vi "test_advanced_Doppler_filtered.vi"() -> ()   [LabVIEW 2009]
doc: "Copyright (C) 2009, Stepan A. Baranov\nweb: http://www.OCTLab.org/\nemail: stepan@baranov.su"
uses:
  OCTLib.dll
panel:
  out "version":string
  out "name":string
  out "error out":errorcluster
  out "max":dbl
  out "min":dbl
  out "cell width":i32
  out "cell height":i32
  out "A-scan size":i32
  out "# of A-scans":i32
  in  "Small/Big":bool
  out "loop #":i32
  out "RSM_STAT time":u32
  out "LabView time":u32
  out "RSM_STAT Array":dbl[][](array[numeric])
  out "LabView Array":dbl[][](array[numeric])
  in  "stop":bool
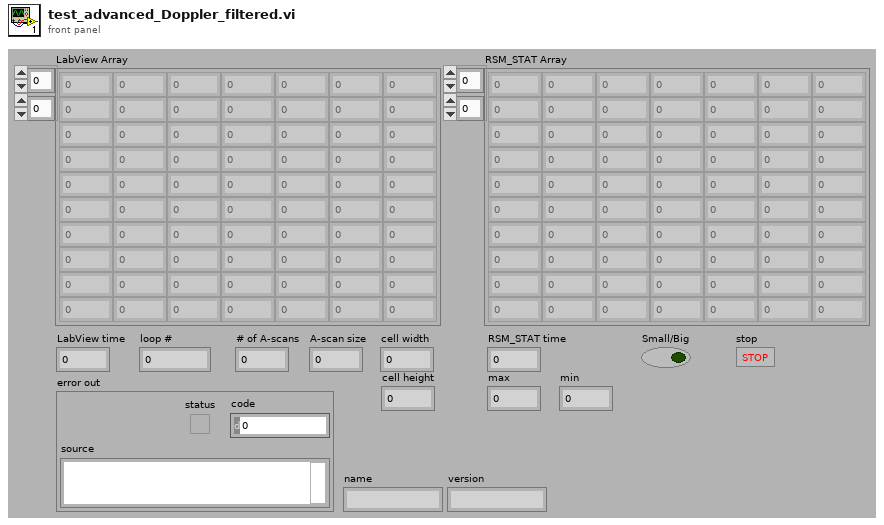
[diagram p1: front panel]
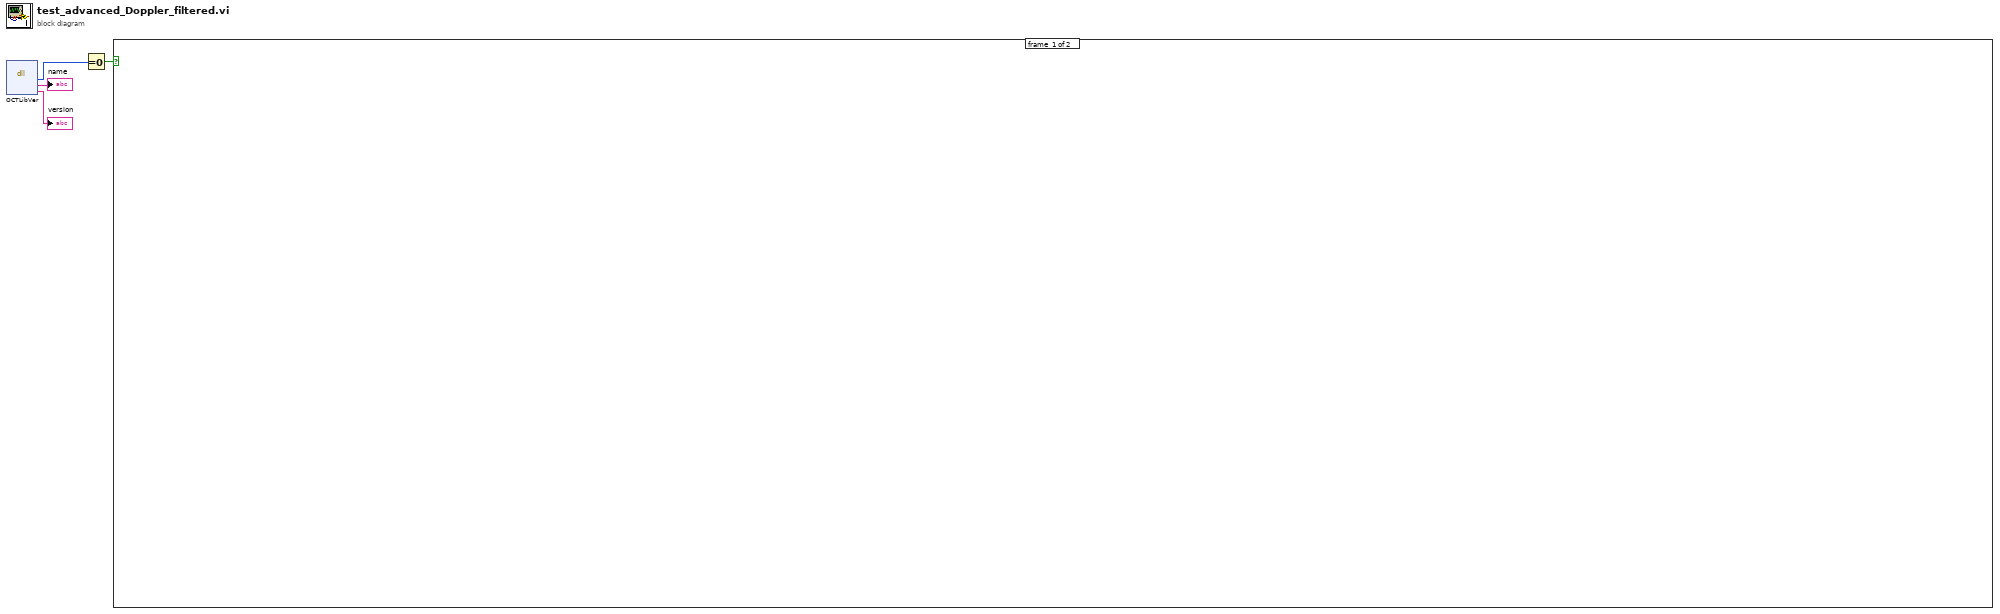
[diagram p0: block diagram]
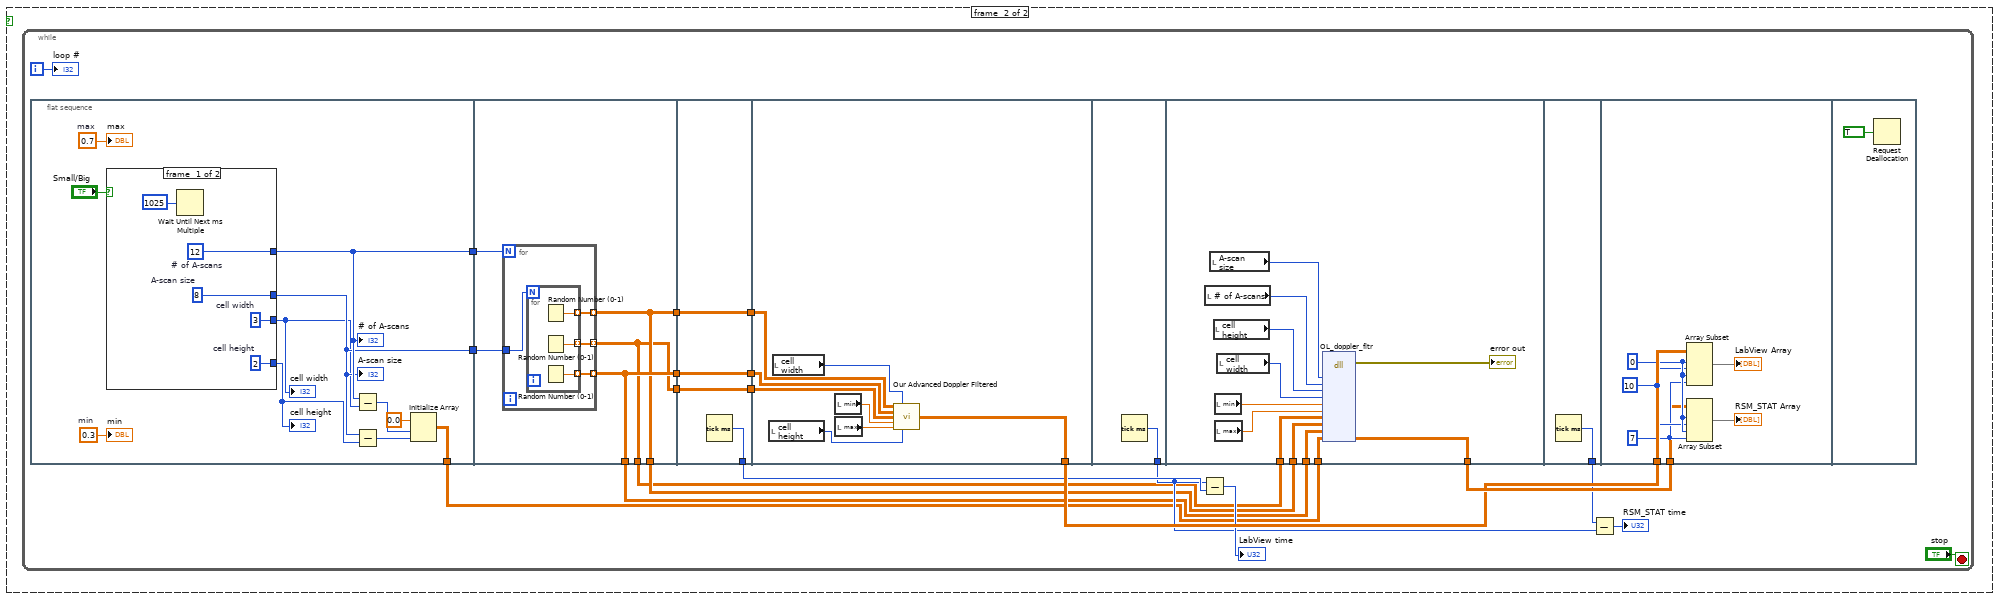
[diagram p2: hidden frame]
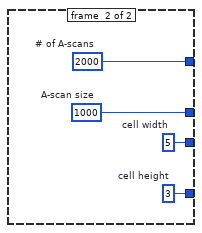
[diagram p3: hidden frame]
diagram:
  n1 = dll-call lib="OCTLib.dll" fn="OCTLibVer"() -> ("status"=w4:i8, "name"=→"name":string, "version"=→"version":string)  [unwired: 5 in, 2 out]
  n2 = Equal To 0?(x=w4) -> (x = 0?=w1:bool)
  n3 = case shown="True" w1 {
    frame #0 {
    }
    frame #1 {
      n4 = while {
        i -> [w17]
        stop <- "stop" stop-if-true
        n5 = flat-sequence {
          tunnel: [w28] -> w13
          tunnel: [w29] -> w12
          tunnel: [w33] -> w8
          tunnel: [w48] -> w16
          tunnel: [w48] -> w14
          tunnel: w13 -> [w50]
          tunnel: w12 -> [w49]
          tunnel: [w47] -> w11
          tunnel: [w47] -> w9
          tunnel: [w46] -> w7
          tunnel: [w46] -> w5
          tunnel: [w61] -> w22
          tunnel: [w60] -> w15
          tunnel: w14 -> [w60]
          tunnel: w11 -> [w58]
          tunnel: [w58] -> w10
          tunnel: w7 -> [w59]
          tunnel: [w59] -> w6
          tunnel: [w69] -> w23
          tunnel: w15 -> [w64]
          tunnel: w10 -> [w66]
          tunnel: w6 -> [w65]
          tunnel: [w70] -> w19
          tunnel: w16 -> [w79]
          tunnel: [w82] -> w24
          tunnel: w9 -> [w78]
          tunnel: w8 -> [w77]
          tunnel: w5 -> [w74]
          tunnel: [w83] -> w20
          tunnel: w24 -> [w84]
          tunnel: w23 -> [w90]
          frame #0 {
            w31 = 0.7  # max
            w32 = 0.3  # min
            n6 = case shown="False" "Small/Big" {
              tunnel: [w40 w44] -> w29
              tunnel: [w41 w45] -> w28
              tunnel: [w38 w43] -> w26
              tunnel: [w37 w42] -> w27
              frame #0 {
                w37 = 2  # cell height
                w38 = 3  # cell width
                w41 = 8  # A-scan size
                w40 = 12  # # of A-scans
                n7 = Wait Until Next ms Multiple(millisecond multiple=u32 1025) -> ()  [unwired: 1 out]
              }
              frame #1 {
                w42 = 3  # cell height
                w43 = 5  # cell width
                w45 = 1000  # A-scan size
                w44 = 2000  # # of A-scans
              }
            }
            "# of A-scans" <- w29
            "A-scan size" <- w28
            "cell height" <- w27
            "cell width" <- w26
            n8 = Subtract(x=w29, y=w26) -> (x-y=w36:i32)
            n9 = Subtract(x=w28, y=w27) -> (x-y=w34:i32)
            n10 = Initialize Array(0.0 ("element"), w36, w34) -> (w33:dbl[][])
            "min" <- w32
            "max" <- w31
          }
          frame #1 {
            n11 = for {
              N: w49 -> [_]
              tunnel: w50 -> [w54]
              tunnel: [w53] -> w48 mode=indexing
              tunnel: [w52] -> w47 mode=indexing
              tunnel: [w51] -> w46 mode=indexing
              n12 = for {
                N: w54 -> [_]
                tunnel: [w57] -> w53 mode=indexing
                tunnel: [w56] -> w52 mode=indexing
                tunnel: [w55] -> w51 mode=indexing
                n13 = Random Number (0-1)() -> (number: 0 to 1=w56:dbl)
                n14 = Random Number (0-1)() -> (number: 0 to 1=w55:dbl)
                n15 = Random Number (0-1)() -> (number: 0 to 1=w57:dbl)
              }
            }
          }
          frame #2 {
            n16 = Tick Count (ms)() -> (millisecond timer value=w61:u32)
          }
          frame #3 {
            n17 = local read "cell height"() -> (w62:i32)
            n18 = local read "cell width"() -> (w63:i32)
            n19 = local read "min"() -> (w68:dbl)
            n20 = local read "max"() -> (w67:dbl)
            n21 = call "Our Advanced Doppler Filtered.vi"("Real Part"=w66, "cell width"=w63, "Imaginary Part"=w64, "intensity"=w65, "min"=w68, "max"=w67, "cell height"=w62) -> ("2D Doppler Image"=w69:dbl[][])  [unwired: 8 in]
          }
          frame #4 {
            n22 = Tick Count (ms)() -> (millisecond timer value=w70:u32)
          }
          frame #5 {
            n23 = local read "# of A-scans"() -> (w80:i32)
            n24 = local read "A-scan size"() -> (w81:i32)
            n25 = local read "cell height"() -> (w72:i32)
            n26 = local read "min"() -> (w75:dbl)
            n27 = local read "max"() -> (w76:dbl)
            n28 = local read "cell width"() -> (w71:i32)
            n29 = dll-call lib="OCTLib.dll" fn="OL_doppler_fltr"("width"=w81, "height"=w80, "cell height"=w72, "cell width"=w71, "min"=w75, "max"=w76, "intensity"=w74, "Re"=w78, "Im"=w79, "data"=w77) -> (error out=→"error out":errorcluster, "data"=w82:dbl[][])  [unwired: 13 in, 1 out]
          }
          frame #6 {
            n30 = Tick Count (ms)() -> (millisecond timer value=w83:u32)
          }
          frame #7 {
            w87 = 10 ("length")
            w86 = 7 ("length")
            w88 = 0 ("index")
            n31 = Array Subset(array=w90, index (row)=w88, length (row)=w87, index (col)=w88, length (col)=w86) -> (→"LabView Array":dbl[][])
            n32 = Array Subset(array=w84, index (row)=w88, length (row)=w87, index (col)=w88, length (col)=w86) -> (→"RSM_STAT Array":dbl[][])
          }
          frame #8 {
            n33 = Request Deallocation(TRUE ("flag")) -> ()
          }
        }
        n34 = Subtract(x=w19, y=w22) -> (x-y=→"LabView time":u32)
        n35 = Subtract(x=w20, y=w19) -> (x-y=→"RSM_STAT time":u32)
        "loop #" <- w17
      }
    }
  }
